vi "Read Flow Rate.vi"(8 "error in (no error)":errorcluster, 11 "CPC in":refnum<class "CPC.lvclass">) -> (0 "error out":errorcluster, 2 "Flow Rate":T1, 3 "CPC out":refnum<class "CPC.lvclass">)   [LabVIEW 2014, in "CPC.lvclass"]
doc: "Get the flow rate that the CPC is currently set for (high or low)."
uses:
  CPC.lvclass
  Controls/3022A/Flow.ctl
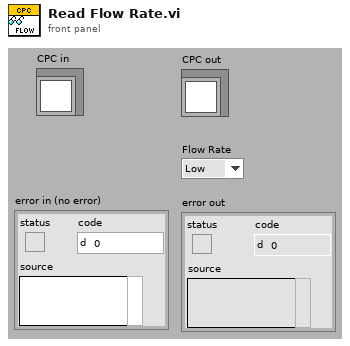
[diagram p1: front panel]
types:
  T1 = typedef "CPC.lvclass/Flow.ctl" = enum16{"Low", "High"}
  T2 = typedef "Flow Rate.ctl" = enum16{"Low", "High"}
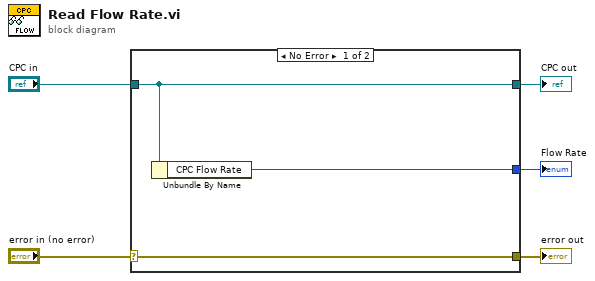
[diagram p0: block diagram]
diagram:
  n1 = case shown="No Error" "error in (no error)" {
    selector: "error in (no error)" -> [w8 w9]
    tunnel: [w8 w9] -> w4
    tunnel: [w7 w10] -> w2
    tunnel: "CPC in" -> [w7 w10]
    tunnel: [w6 _] -> w1
    frame No Error {
      n2 = Unbundle By Name(w7) -> ("CPC Flow Rate"=w6:T2)
    }
    frame Error {
    }
  }
  "error out" <- w4
  "CPC out" <- w2
  "Flow Rate" <- w1
